vi "On Recompile Action VI Name.vi"(11 "CD Template in":refnum<class "NIVS_PPL_Inline HW Interface (Inline-Async).lvclass">) -> (2 "On Recompile Action VI Name":string)   [LabVIEW 2020, in "NIVS_PPL_Inline HW Interface (Inline-Async).lvclass"]
uses:
  NIVS_PPL_Inline HW Interface (Inline-Async).lvclass
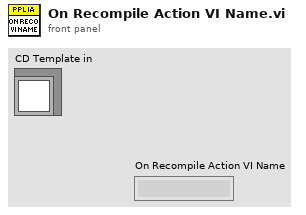
[diagram p1: front panel]
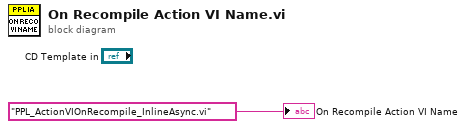
[diagram p0: block diagram]
diagram:
  "On Recompile Action VI Name" <- "PPL_ActionVIOnRecompile_InlineAsync.vi" ("On Recompile Action VI Name")
